vi "Delete Object.vi"(4 "Region":T1, 6 "Auth Device Data":T3, 7 "Version ID":string, 8 "error in (no error)":errorcluster, 9 "Bucket":string, 10 "Object Path":string) -> (0 "error out":errorcluster, 3 "Versioning Data":T2)   [LabVIEW 2015, in "LV Interface for Amazon S3.lvlib"]
doc: "The operation <B>removes the null version</B> (if there is one) <B>of an object and inserts a delete marker</B>, which becomes the latest version of the object. If there isn't a null version, Amazon S3 does not remove any objects."
uses:
  LV Interface for Amazon S3.lvlib
  Typedefs/AMZ_S3_Auth Device Data.ctl
  Typedefs/AMZ_S3_API_Delete Object with Versioning Result.ctl
  Typedefs/AMZ_S3_LocationConstraint.ctl
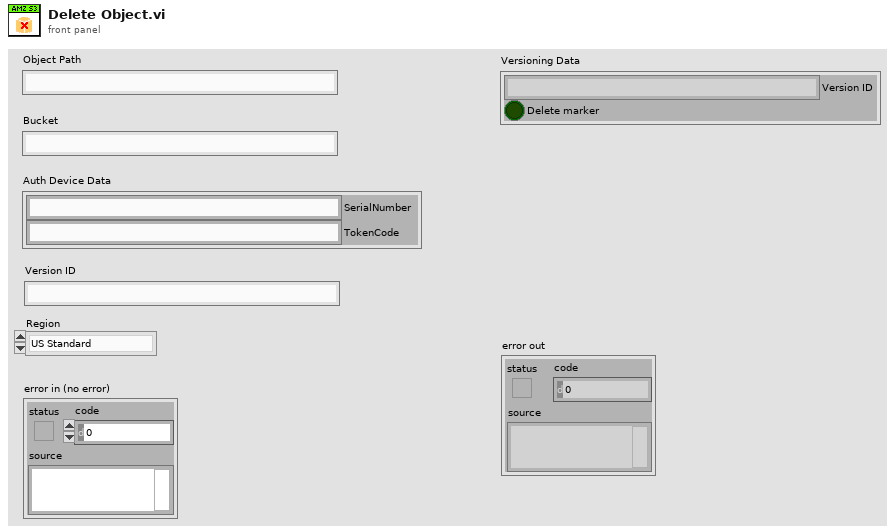
[diagram p1: front panel]
types:
  T1 = typedef "LV Interface for Amazon S3.lvlib/AMZ_S3_LocationConstraint.ctl" = enum16{"US Standard", "us-east-2", "us-west-1", "us-west-2", "ap-northeast-1", "ap-northeast-2", "ap-southeast-1", "ap-southeast-2", "ca-central-1", "eu-central-1", "eu-west-1", "eu-west-2", "sa-east-1"}
  T2 = typedef "LV Interface for Amazon S3.lvlib/AMZ_S3_API_Delete Object with Versioning Result.ctl" = cluster{"Version ID":string, "Delete marker":bool}
  T3 = typedef "LV Interface for Amazon S3.lvlib/AMZ_S3_Auth Device Data.ctl" = cluster{"SerialNumber":string, "TokenCode":string}
  T4 = typedef "LV Interface for Amazon S3.lvlib/AMZ_S3_HTTP Header-Value pair.ctl" = cluster{"Header":string, "Value":string}
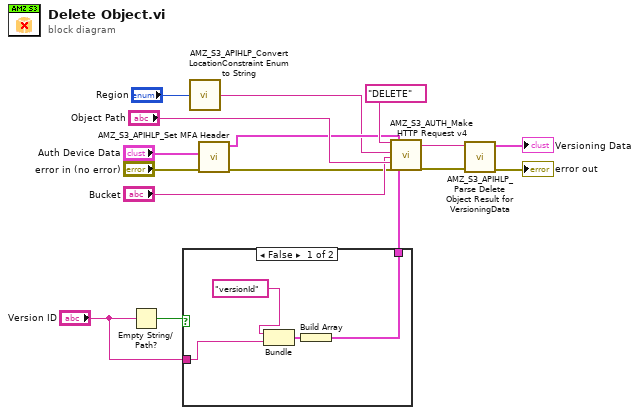
[diagram p0: block diagram]
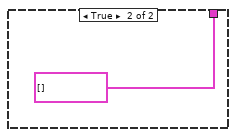
[diagram p2: hidden frame]
diagram:
  n1 = Empty String/Path?(string/path="Version ID") -> (empty?=w5:bool)
  n2 = case shown="False" w5 {
    tunnel: [w17 cluster{"item":string, "value":string}[] [] ("request parameters")] -> w4
    tunnel: "Version ID" -> [w20 _]
    frame False {
      n3 = Bundle("versionId", "Version ID"=w20) -> (w18:cluster{string, "Version ID":string})  [unwired: 1 in]
      n4 = Build Array(w18) -> (w17:cluster{string, "Version ID":string}[])
    }
    frame True {
    }
  }
  n5 = call "AMZ_S3_APIHLP_Convert LocationConstraint Enum to String.vi"("Location"="Region") -> ("Location String"=w1:string)  [unwired: 4 in]
  n6 = call "AMZ_S3_APIHLP_Set MFA Header.vi"("error in (no error)"="error in (no error)", "Auth device data"="Auth Device Data") -> ("error out"=w8:errorcluster, "HTTP Headers"=w9:T4[])  [unwired: 7 in, 1 out]
  n7 = call "AMZ_S3_AUTH_Make HTTP Request v4.vi"("HTTP-Verb"="DELETE", "Region"=w1, "Bucket"="Bucket", "Object Key"="Object Path", "error in"=w8, "request headers"=w9, "request parameters"=w4) -> ("response headers"=w6:string, "error out"=w7:errorcluster)  [unwired: 9 in, 2 out]
  n8 = call "AMZ_S3_APIHLP_Parse Delete Object Result for VersioningData.vi"("error in (no error)"=w7, "Response header"=w6) -> ("error out"=→"error out":errorcluster, "Versioning Data"=→"Versioning Data":T2)  [unwired: 8 in]
